vi "Convert Span Size to Time.vi"(10 "Expected Total Data Size (Bytes/sec)":dbl, 11 "File Log Specification In":T1={"Directory"=path "", "Groups"=[], "Buffer Size"=0, "Properties"=[], "Pretrigger"=FALSE, "Name"="", "Timestamp"=FALSE, "Error"=0, "Auto Open"=FALSE, "File Node Ref"=18446744073709551615, "Archive"=FALSE, "Archive Directory"=path "", "Segment Files"=FALSE, "Segment Files By"=enum."Size", "Segment Size"=100000} {"File Node Ref" format="%.0x"}) -> (3 "File Log Specification Out":T1={"Directory"=path "", "Groups"=[], "Buffer Size"=0, "Properties"=[], "Pretrigger"=FALSE, "Name"="", "Timestamp"=FALSE, "Error"=0, "Auto Open"=FALSE, "File Node Ref"=18446744073709551615, "Archive"=FALSE, "Archive Directory"=path "", "Segment Files"=FALSE, "Segment Files By"=enum."Size", "Segment Size"=100000} {"File Node Ref" format="%.0x"})   [LabVIEW 2018, in "Embedded Data Logger Engine.lvlib"]
uses:
  Embedded Data Logger Engine.lvlib
  File Logging Specification.ctl
  Group Logging Specification.ctl
  Group Buffer Data.ctl
  Property Specification.ctl
  <vilib>/NI Veristand/Custom Device API/Custom Device Item Ref.ctl
  Shared/Segment Files By.ctl
  Shared/Embedded Data Logger Shared.lvlib
  <vilib>/NI Veristand/Custom Device API/Custom Device API.lvlib
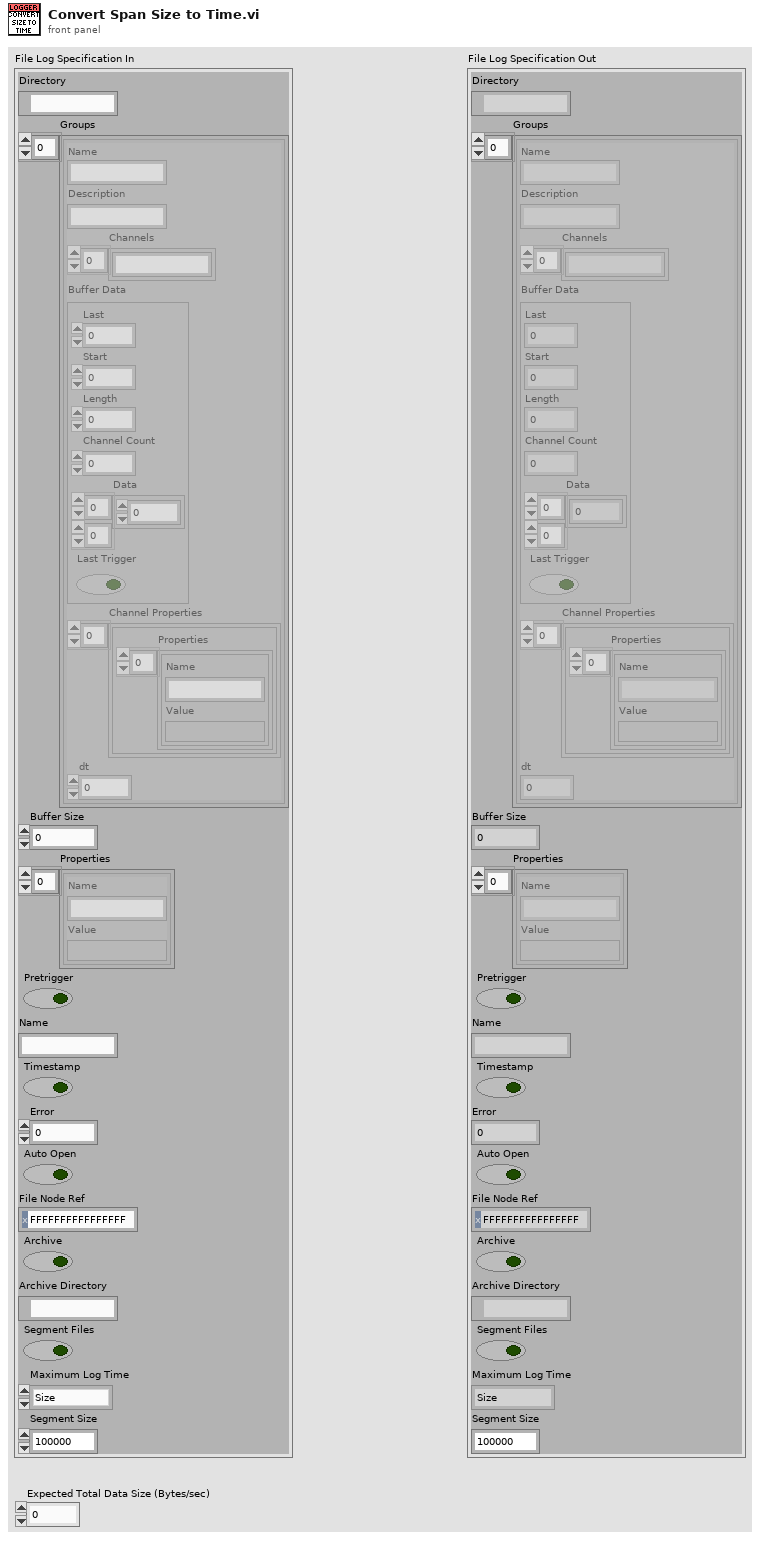
[diagram p1: front panel]
types:
  T1 = typedef "Embedded Data Logger Engine.lvlib/File Logging Specification.ctl" = cluster{"Directory":path, "Groups":T2[], "Buffer Size":i32, "Properties":T4[], "Pretrigger":bool, "Name":string, "Timestamp":bool, "Error":i32, "Auto Open":bool, "File Node Ref":T5, "Archive":bool, "Archive Directory":path, "Segment Files":bool, "Segment Files By":T6, "Segment Size":u32}
  T2 = typedef "Embedded Data Logger Engine.lvlib/Group Logging Specification.ctl" = cluster{"Name":string, "Description":string, "Channels":string[], "Buffer Data":T3, "Channel Properties":cluster{"Properties":T4[]}[], "dt":dbl}
  T3 = typedef "Embedded Data Logger Engine.lvlib/Group Buffer Data.ctl" = cluster{"Last":i32, "Start":i32, "Length":i32, "Channel Count":i32, "Data":dbl[][], "Last Trigger":bool}
  T4 = typedef "Embedded Data Logger Engine.lvlib/Property Specification.ctl" = cluster{"Name":string, "Value":variant}
  T5 = typedef "Custom Device API.lvlib/Custom Device Item Ref.ctl" = u64
  T6 = typedef "Embedded Data Logger Shared.lvlib/Segment Files By.ctl" = enum16{"Time", "Size"}
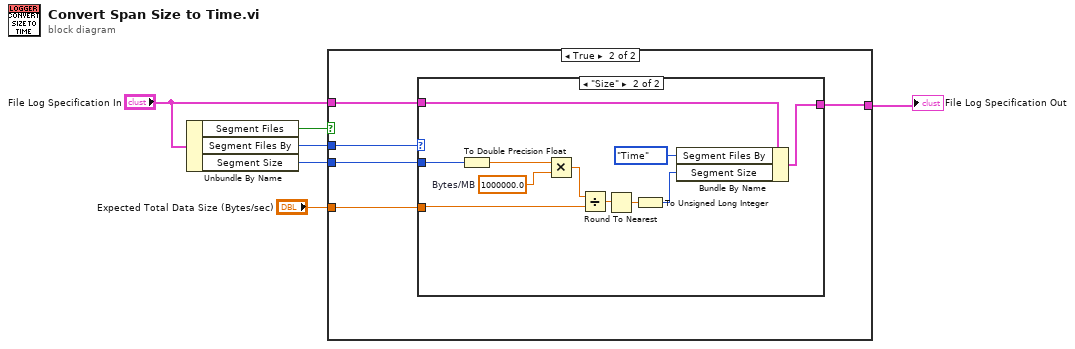
[diagram p0: block diagram]
diagram:
  n1 = Unbundle By Name("File Log Specification In") -> ("Segment Files"=w5:bool, "Segment Files By"=w6:T6, "Segment Size"=w4:u32)
  n2 = case shown="True" w5 {
    tunnel: w6 -> [_ w12]
    tunnel: w4 -> [_ w11]
    tunnel: "File Log Specification In" -> [w7 w10]
    tunnel: "Expected Total Data Size (Bytes/sec)" -> [_ w9]
    tunnel: [w7 w8] -> w2
    frame False {
    }
    frame True {
      n3 = case shown="\"Size\"" w12 {
        tunnel: w11 -> [_ w24]
        tunnel: w10 -> [w13 w19]
        tunnel: w9 -> [_ w20]
        tunnel: [w13 w17] -> w8
        frame "Time", Default {
        }
        frame "Size" {
          w22 = 1000000.0  # Bytes/MB
          n4 = To Double Precision Float(number=w24) -> (double precision float=w23:dbl)
          n5 = Multiply(x=w23, y=w22) -> (x*y=w21:dbl)
          n6 = Divide(x=w21, y=w20) -> (x/y=w15:dbl)
          n7 = Round To Nearest(number=w15) -> (nearest integer value=w14:dbl)
          n8 = To Unsigned Long Integer(number=w14) -> (unsigned 32bit integer=w16:u32)
          n9 = Bundle By Name(cluster=w19, "Segment Files By"=Segment_Files_By."Time", "Segment Size"=w16) -> (w17:T1)
        }
      }
    }
  }
  "File Log Specification Out" <- w2
